vi "CMI ckd2 Write and Read.vi"(8 "error in":errorcluster, 9 "read byte count (0 - no receive)":u32, 10 "command":string, 11 "session":T1) -> (0 "error out":errorcluster, 2 "read buffer":string, 3 "session out":T1)   [LabVIEW 2020, in "AWG.lvlib"]
doc: "Flushes RX buffer, sends command, waits for answer if non-zero read count is set."
uses:
  AWG.lvlib
  CMI ckd2 Session.ctl
  CMI ckd2 Source Mode.ctl
  <vilib>/Instr/_visa.llb/VISA Flush IO Buffer Mask.ctl
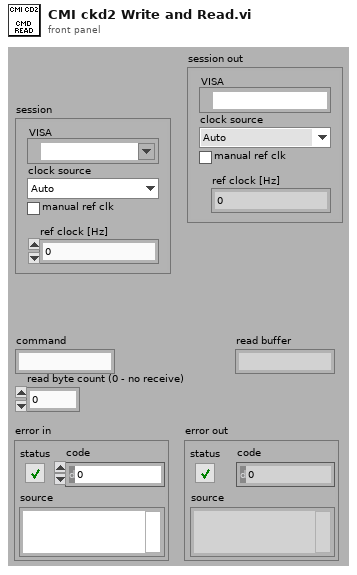
[diagram p1: front panel]
types:
  T1 = typedef "AWG.lvlib/CMI ckd2 Session.ctl" = cluster{"VISA":refnum<visa-resource-name>, "clock source":T2, "manual ref clk":bool, "ref clock [Hz]":dbl}
  T2 = typedef "AWG.lvlib/CMI ckd2 Source Mode.ctl" = enum16{"Auto", "LF clock", "HF clock", "Internal"}
  T3 = typedef "VISA Flush IO Buffer Mask.ctl" = u16
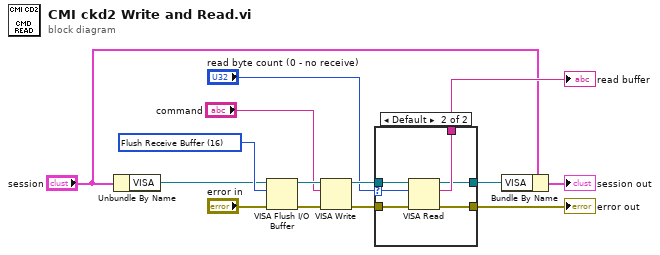
[diagram p0: block diagram]
diagram:
  w13 = T3 16 items=["Flush Receive Buffer"=16, "Write Transmit Buffer to Device"=32, "Flush Receive Buffer (No I/O)"=64, "Flush Transmit Buffer"=128] ("Mask")
  n1 = Unbundle By Name("session") -> ("VISA"=w5:refnum<visa-resource-name>)
  n2 = VISA Flush I/O Buffer(VISA resource name=w5, mask (16)=w13, error in (no error)="error in") -> (VISA resource name out=w11:refnum<visa-resource-name>, error out=w12:errorcluster)
  n3 = VISA Write(VISA resource name=w11, write buffer="command", error in (no error)=w12) -> (VISA resource name out=w8:refnum<visa-resource-name>, error out=w9:errorcluster)  [unwired: 1 out]
  n4 = case shown="Default" "read byte count (0 - no receive)" {
    selector: "read byte count (0 - no receive)" -> [_ w17]
    tunnel: w9 -> [w16 w22]
    tunnel: w8 -> [w15 w21]
    tunnel: [w16 w20] -> w7
    tunnel: [_ w19] -> w6
    tunnel: [w15 w18] -> w3
    frame 0 {
    }
    frame Default {
      n5 = VISA Read(VISA resource name=w21, byte count=w17, error in (no error)=w22) -> (VISA resource name out=w18:refnum<visa-resource-name>, read buffer=w19:string, error out=w20:errorcluster)  [unwired: 1 out]
    }
  }
  "error out" <- w7
  "read buffer" <- w6
  n6 = Bundle By Name(cluster="session", "VISA"=w3) -> (→"session out":T1)
